vi "WF.vi"() -> ()   [LabVIEW 2013]
uses:
  <vilib>/Utility/error.llb/DialogType.ctl
  <vilib>/DAQmx/write.llb/DAQmx Write (Analog 1D DBL NChan 1Samp).vi
  <vilib>/DAQmx/create/channels.llb/DAQmx Create Channel (AO-Voltage-Basic).vi
  <vilib>/DAQmx/miscellaneous.llb/DAQmx Fill In Error Info.vi
panel:
  in  "曝光时间/ms":dbl
  in  "Array":dbl[][](array[numeric])
  in  "Physical Channel(s)":tag[](array[tag])=["cDAQ1Mod1/ao0", "cDAQ1Mod1/ao2", "cDAQ1Mod1/ao1", "cDAQ1Mod1/ao15", "cDAQ1Mod1/ao14", "cDAQ1Mod1/ao13"]
  # "宽场相机触发"
  # "488LED"
  # "561LED"
  # "637LED"
  # "明场开"
  # "明场关"
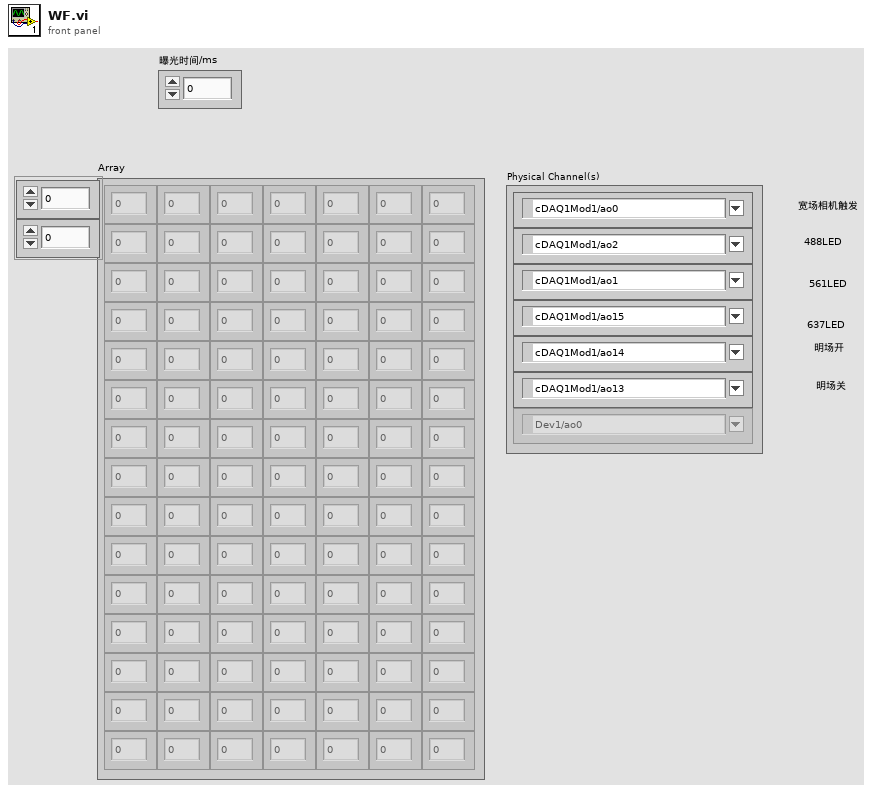
[diagram p1: front panel]
types:
  T1 = typedef "DialogType.ctl" = u16
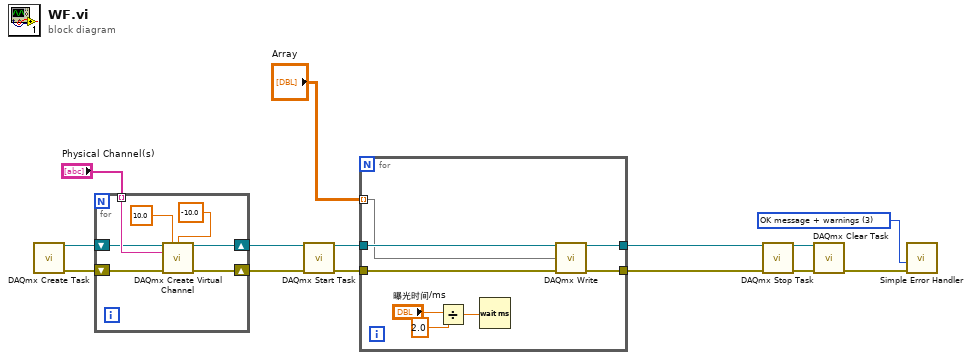
[diagram p0: block diagram]
diagram:
  w9 = T1 3 items=["no dialog", "OK message", "continue or stop message", "OK message + warnings", "continue/stop + warnings"] ("type of dialog (OK msg:1)")
  n1 = call <vilib>:"DAQmx Create Task.vi"() -> ("task out"=w8:refnum<k21>, "error out"=w7:errorcluster)  [unwired: 14 in]
  n2 = for {
    shift-right: [w21] -> w13
    shift-left: w8 -> [w16]
    shift-right: [w20] -> w12
    shift-left: w7 -> [w15]
    tunnel: "Physical Channel(s)" -> [w17] mode=indexing
    n3 = call-poly <vilib>:"DAQmx Create Virtual Channel.vi"("task in"=w16, "maximum value"=10.0, "minimum value"=-10.0, "physical channels"=w17, "error in"=w15) -> ("task out"=w21:refnum<k21>, "error out"=w20:errorcluster)  [unwired: 9 in]
  }
  n4 = call <vilib>:"DAQmx Start Task.vi"("task/channels in"=w13, "error in"=w12) -> ("task out"=w5:refnum<k21>, "error out"=w4:errorcluster)  [unwired: 12 in]
  n5 = for {
    tunnel: w5 -> [w29]
    tunnel: w4 -> [w28]
    tunnel: [w27] -> w3
    tunnel: [w26] -> w2
    tunnel: "Array" -> [w22] mode=indexing
    n6 = Divide(x="曝光时间/ms", y=2.0) -> (x/y=w23:dbl)
    n7 = Wait (ms)(milliseconds to wait=w23) -> ()  [unwired: 1 out]
    n8 = call-poly <vilib>:"DAQmx Write.vi"("task/channels in"=w29, "data"=w22, "error in"=w28) -> ("task out"=w26:refnum<k21>, "error out"=w27:errorcluster)  [unwired: 10 in, 1 out]
  }
  n9 = call <vilib>:"DAQmx Stop Task.vi"("task/channels in"=w2, "error in"=w3) -> ("task out"=w11:refnum<k21>, "error out"=w10:errorcluster)  [unwired: 12 in]
  n10 = call <vilib>:"DAQmx Clear Task.vi"("task in"=w11, "error in"=w10) -> ("error out"=w14:errorcluster)  [unwired: 13 in]
  n11 = call <vilib>:"Simple Error Handler.vi"("type of dialog (OK msg:1)"=w9, "error in (no error)"=w14) -> ()  [unwired: 3 in, 5 out]
